vi "Get Subtype Description.vi"(8 "error in (no error)":errorcluster, 11 "Timing Action in":refnum<class "Timing Action.lvclass">) -> (0 "error out":errorcluster, 2 "Subtype Description":string, 3 "Timing Action out":refnum<class "Timing Action.lvclass">)   [LabVIEW 2020, in "MacroAssert.lvlib" / "Timing Action.lvclass"]
uses:
  Timing Action.lvclass
  Timing Action.lvclass/Timing Action.ctl
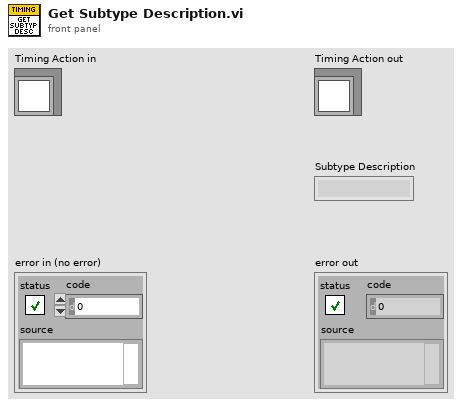
[diagram p1: front panel]
types:
  T1 = typedef "MacroAssert.lvlib/Timing Action.lvclass/Timing Action Type.ctl" = enum16{"Wait", "Wait Until"}
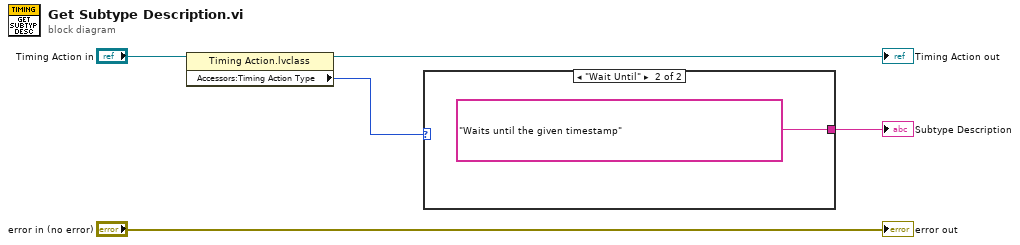
[diagram p0: block diagram]
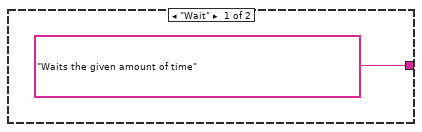
[diagram p2: hidden frame]
diagram:
  n1 = property class="Timing Action.lvclass"(reference="Timing Action in") -> (reference out=→"Timing Action out":refnum<class "Timing Action.lvclass">, "Accessors:Timing Action Type"=w5:T1)  [unwired: 1 in, 1 out]
  n2 = case shown="\"Wait Until\"" w5 {
    tunnel: ["Waits the given amount of time" "Waits until the given timestamp"] -> w2
    frame "Wait" {
    }
    frame "Wait Until" {
    }
  }
  "Subtype Description" <- w2
  "error out" <- "error in (no error)"
